vi "debug.vi"(9 "压力点个数":dbl, 10 "检定次数":dbl) -> (6 "I":dbl[](array[numeric]), 8 "A":dbl[](array[numeric]))   [LabVIEW 2017]
panel:
  in  "产品编号":string[](array[string])
  in  "参数计算":bool
  in  "加载参数":bool
  in  "保存参数":bool
  in  "偏置增益调试文件名":string="2022917_1556_70.0"
  in  "补偿电阻调试文件名":string="2022917_1556_70.0"
  in  "控制板调试":bool
  out "Rp":dbl[](array[numeric])
  out "Rs":dbl[](array[numeric])
  in  "退出":bool
  in  "行程测试":bool
  out "Rx":dbl[](array[numeric])
  out "Rf":dbl[](array[numeric])
  in  "偏置增益计算":bool
  in  "补偿电阻计算":bool
  out "理论曲线":string
  in  "理论偏置 b":dbl=200.0
  in  "理论放大 K":dbl=287.5
  out "Vx":dbl[](array[numeric])
  in  "Radj1":dbl[](array[numeric])
  in  "RG":dbl[](array[numeric])
  in  "R5-1":dbl[](array[numeric])
  in  "R4-6":dbl[](array[numeric])
  in  "R5-6":dbl[](array[numeric])
  in  "R5-5":dbl[](array[numeric])
  in  "R5-4":dbl[](array[numeric])
  in  "R4-4":dbl[](array[numeric])
  in  "R3-2":dbl[](array[numeric])
  in  "R3-1":dbl[](array[numeric])
  in  "数据":dbl[][](array[numeric])=[[199.921, 4.0, 7.8325, 4.0, -2.844e-06, -3.3e-06, -3.109e-06, -3.045e-06, -2.897e-06, 1.0, 0.0], [299.9351, 4.0, 7.8338, 1.0, -3.491e-06, -2.918e-06, -3.332e-06, -2.78e-06, -3.204e-06, 0.0, 0.0], [399.96, 4.0, 7.8346, -3.12e-06, -3.289e-06, -2.96e-06, -3.141e-06, -3.385e-06, -2.844e-06, 0.0, 0.0], [400.0285, -4.0, 7.8346, 0.0, -3.342e-06, -3.162e-06, -3.194e-06, -3.056e-06, -3.194e-06, 0.0, 0.0], [300.0653, -4.0, 7.8332, -3.342e-06, -3.321e-06, -3.013e-06, -3.311e-06, -3.3e-06, -3.162e-06, 0.0, 0.0], [200.0595, -4.0, 7.8346, -2.907e-06, -3.194e-06, -3.257e-06, -3.204e-06, -3.077e-06, -2.971e-06, 0.0, 0.0], [199.9466, 4.0, 8.8568, 5.0, -3.353e-06, -3.799e-06, -3.565e-06, -3.746e-06, -3.374e-06, 0.0, 0.0], [299.95, 4.0, 8.8574, -3.311e-06, -3.502e-06, -3.364e-06, -3.618e-06, -3.12e-06, -3.406e-06, 0.0, 0.0], [399.8962, 4.0, 8.8567, -3.756e-06, -3.83e-06, -3.427e-06, -3.597e-06, -3.777e-06, -3.576e-06, 0.0, 0.0], [399.9835, -4.0, 8.8567, 0.0, -3.289e-06, -3.12e-06, -3.502e-06, -3.427e-06, -3.353e-06, 0.0, 0.0], [299.9459, -4.0, 8.8552, -3.512e-06, -3.65e-06, -3.809e-06, -3.48e-06, -3.3e-06, -3.767e-06, 0.0, 0.0], [199.9841, -4.0, 8.8564, -3.629e-06, -3.608e-06, -3.767e-06, -3.639e-06, -3.417e-06, -3.406e-06, 0.0, 0.0], [200.0, 4.0, 0.0, 1.0, 0.0, 0.0, 0.0, 0.0, 0.0, 0.0, 0.0], [300.0, 4.0, 0.0, 2.0, 0.0, 0.0, 0.0, 0.0, 0.0, 0.0, 0.0], [400.0, 4.0, 0.0, 3.0, 0.0, 0.0, 0.0, 0.0, 0.0, 0.0, 0.0], [400.0, -4.0, 0.0, 20.0, 0.0, 0.0, 0.0, 0.0, 0.0, 0.0, 0.0], [300.0, -4.0, 0.0, 5.0, 0.0, 0.0, 0.0, 0.0, 0.0, 0.0, 0.0], [200.0, -4.0, 0.0, 6.0, 0.0, 0.0, 0.0, 0.0, 0.0, 0.0, 0.0], [200.0, 0.0, 0.0, 7.0, 0.0, 0.0, 0.0, 0.0, 0.0, 0.0, 0.0], [300.0, 0.0, 0.0, 8.0, 0.0, 0.0, 0.0, 0.0, 0.0, 0.0, 0.0], [400.0, 0.0, 0.0, 9.0, 0.0, 0.0, 0.0, 0.0, 0.0, 0.0, 0.0], [400.0, -7.0, 0.0, 10.0, 0.0, 0.0, 0.0, 0.0, 0.0, 0.0, 0.0], [300.0, -7.0, 0.0, 11.0, 0.0, 0.0, 0.0, 0.0, 0.0, 0.0, 0.0], [200.0, -7.0, 0.0, 12.0, 0.0, 0.0, 0.0, 0.0, 0.0, 0.0, 0.0], [0.0, 0.0, 0.0, 13.0, 0.0, 0.0, 0.0, 0.0, 0.0, 0.0, 0.0], [0.0, 0.0, 0.0, 14.0, 0.0, 0.0, 0.0, 0.0, 0.0, 0.0, 0.0], [0.0, 0.0, 0.0, 15.0, 0.0, 0.0, 0.0, 0.0, 0.0, 0.0, 0.0], [0.0, -7.0, 0.0, 16.0, 0.0, 0.0, 0.0, 0.0, 0.0, 0.0, 0.0], [0.0, -7.0, 0.0, 17.0, 0.0, 0.0, 0.0, 0.0, 0.0, 0.0, 0.0], [0.0, -7.0, 0.0, 18.0, 0.0, 0.0, 0.0, 0.0, 0.0, 0.0, 0.0], [0.0, 0.0, 0.0, 19.0, 0.0, 0.0, 0.0, 0.0, 0.0, 0.0, 0.0], [0.0, 0.0, 0.0, 20.0, 0.0, 0.0, 0.0, 0.0, 0.0, 0.0, 0.0], [0.0, 0.0, 0.0, 21.0, 0.0, 0.0, 0.0, 0.0, 0.0, 0.0, 0.0], [0.0, -7.0, 0.0, 22.0, 0.0, 0.0, 0.0, 0.0, 0.0, 0.0, 0.0], [0.0, -7.0, 0.0, 23.0, 0.0, 0.0, 0.0, 0.0, 0.0, 0.0, 0.0], [0.0, -7.0, 0.0, 24.0, 0.0, 0.0, 0.0, 0.0, 0.0, 0.0, 0.0], [0.0, 0.0, 0.0, 25.0, 0.0, 0.0, 0.0, 0.0, 0.0, 0.0, 0.0], [0.0, 0.0, 0.0, 26.0, 0.0, 0.0, 0.0, 0.0, 0.0, 0.0, 0.0], [0.0, 0.0, 0.0, 27.0, 0.0, 0.0, 0.0, 0.0, 0.0, 0.0, 0.0]]
  # "多通道 传感器调试系统"
  # "结果计算"
  # "参数设置  单位（Ω）"
  # "1"
  # "2"
  # "3"
  # "4"
  # "5"
  # "6"
  # "7"
  # "8"
  # "9"
  # "10"
  # "1"
  # "2"
  # "3"
  # "4"
  # "5"
  # "6"
  # "7"
  # "8"
  # "9"
  # "10"
  # "传感器编号"
  # "A"
  # "R3-1"
  # "I(mA)"
  # "R3-2"
  # "Vx(V)"
  # "R4-4"
  # "R4-6"
  # "Rs(kΩ)"
  # "R5-1"
  # "Rp(MΩ)"
  # "R5-4"
  # "R5-5"
  # "Rf(kΩ)"
  # "R5-6"
  # "Rx(Ω)"
  # "RG"
  # "Radj1"
  # "注意：\n调试系统，支持可变个传感器调试，不必连接10个。支持个数范围（1-无穷大）\n调试前，请参照调试规范，预先筛选安装并测量上述每个电阻的电阻值。\n在计算 补偿电阻 与 偏置增益 前 请按照说明规范设置参数，并进行相应的自动化测试。\n计算 补偿电阻 与 偏置增益 请输入正确的信息。如需 系统自动获取，请置空相应输入信息。\n补偿电阻调试时，请在低温（-40℃）与高温（70℃）两个温度点进行，压力点设置为常压、15MPa两个点。\n偏置增益调试时、请在常温下进行6个压力点(20KPa, 100KPa, 1000KPa, 5000KPa, 10000KPa, 15000KPa)的测量。"
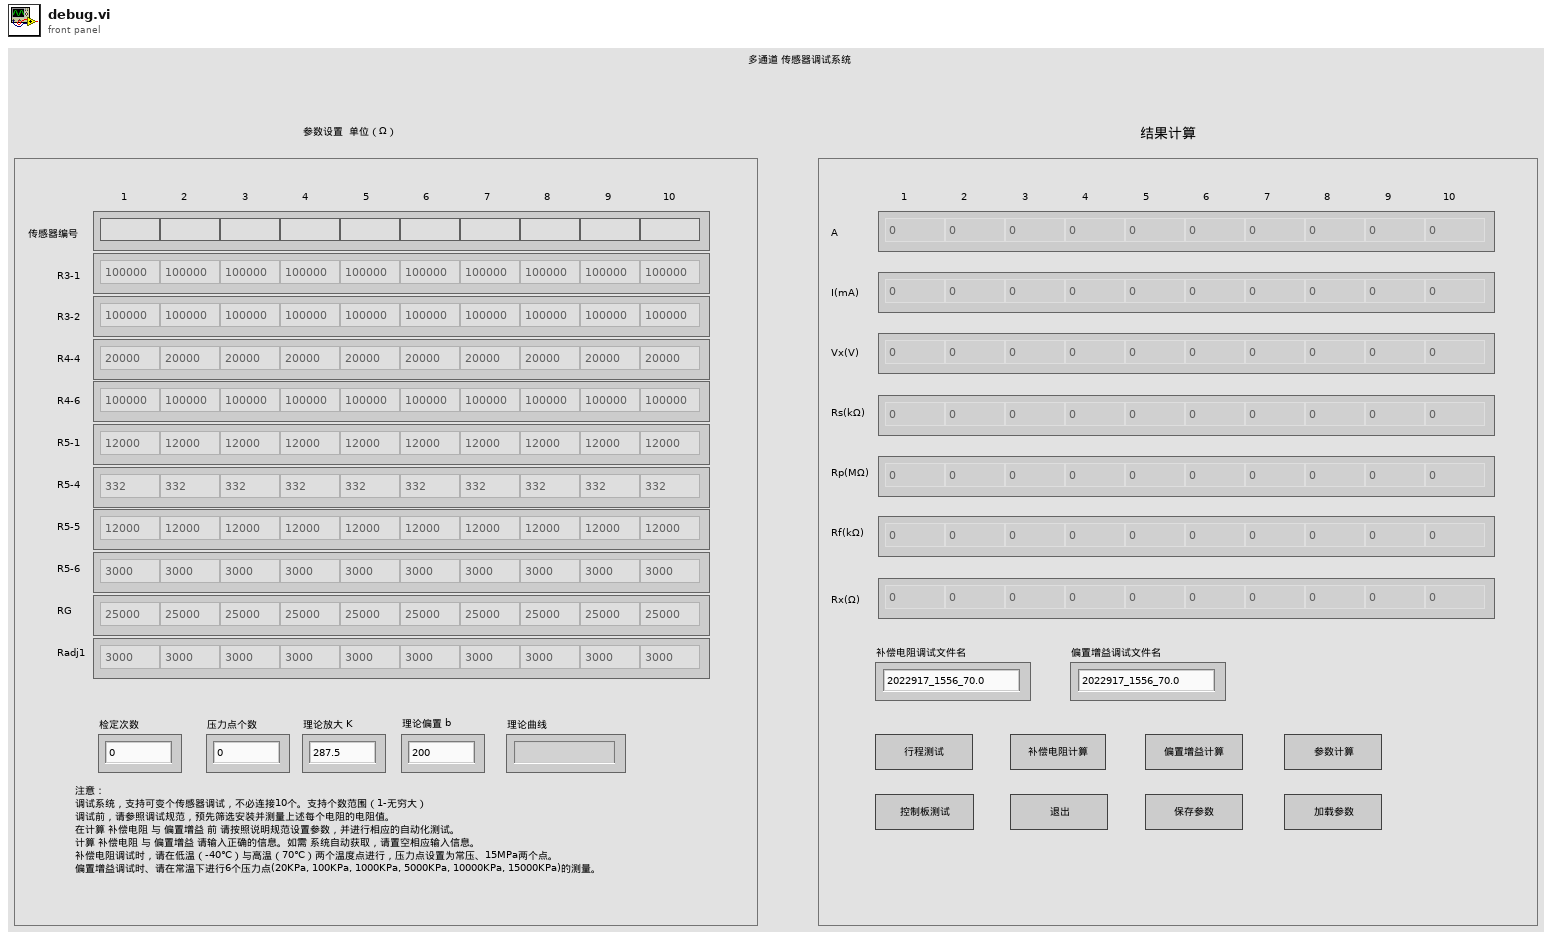
[diagram p1: front panel]
types:
  T1 = enum32{"Invalid", "Standard", "Closed", "Hidden", "Minimized", "Maximized"}
  T2 = enum16{"open", "replace", "create", "open or create", "replace or create", "replace or create with confirmation"}
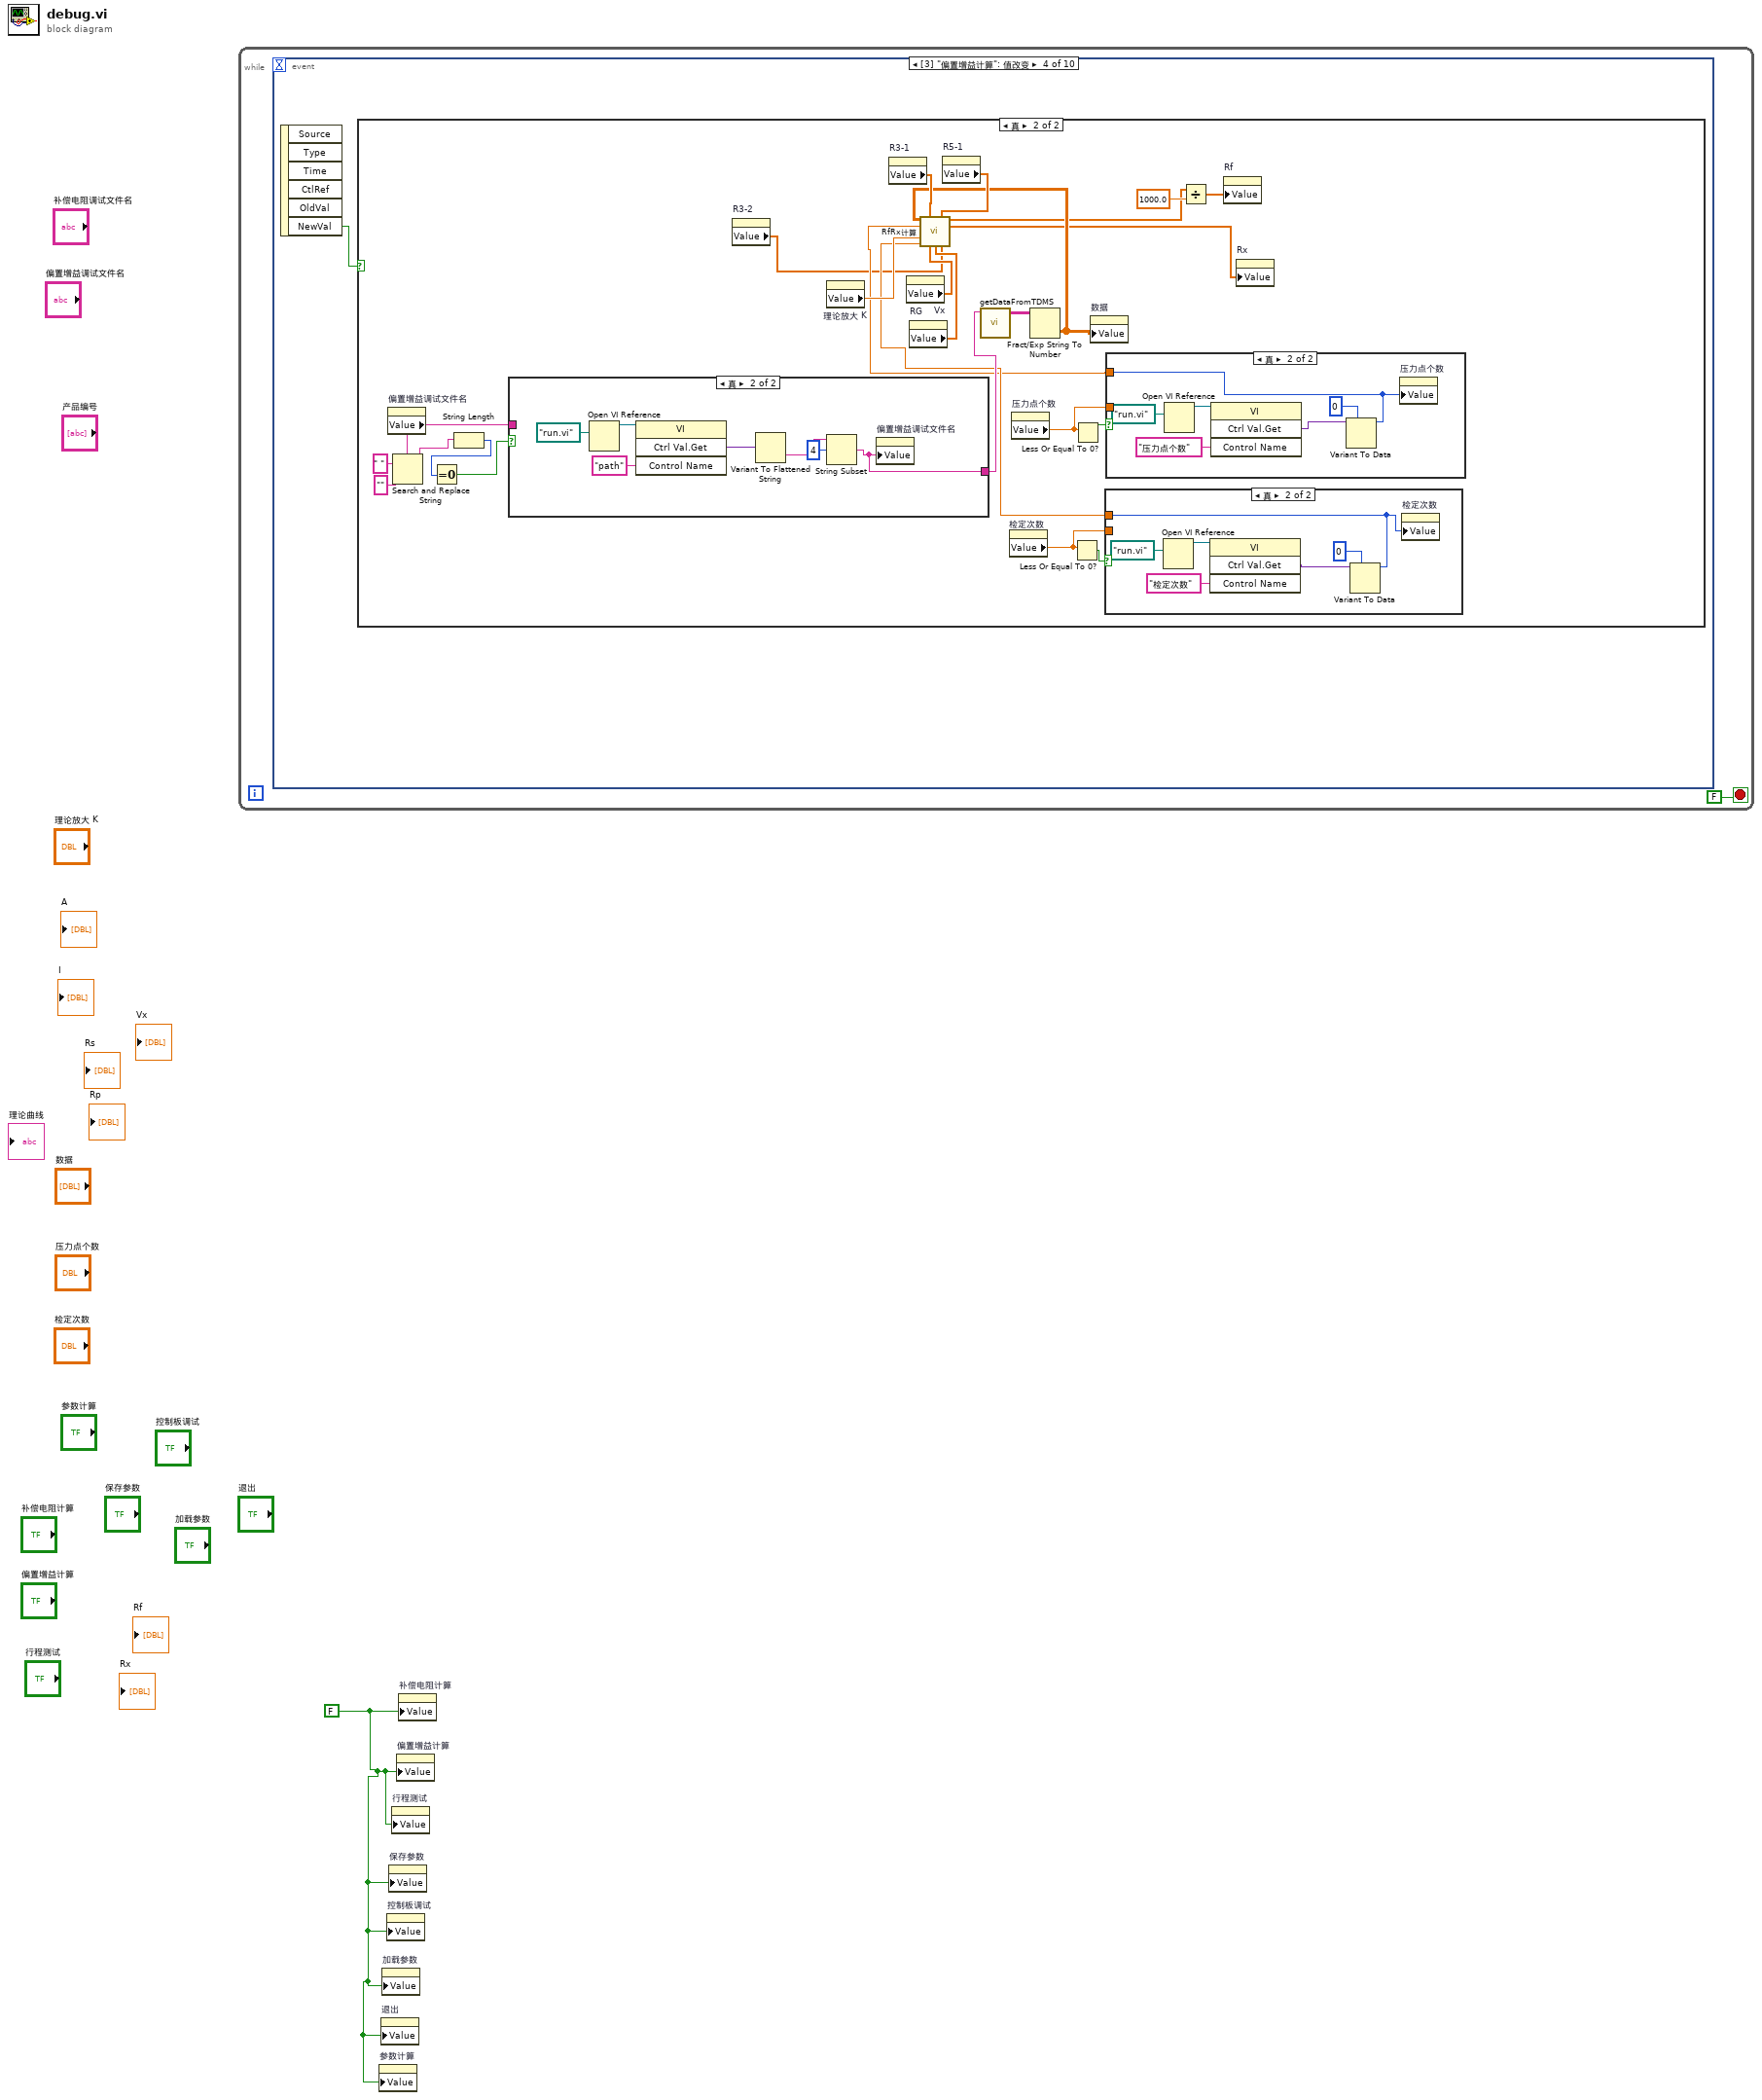
[diagram p0: block diagram]
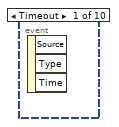
[diagram p2: hidden frame]
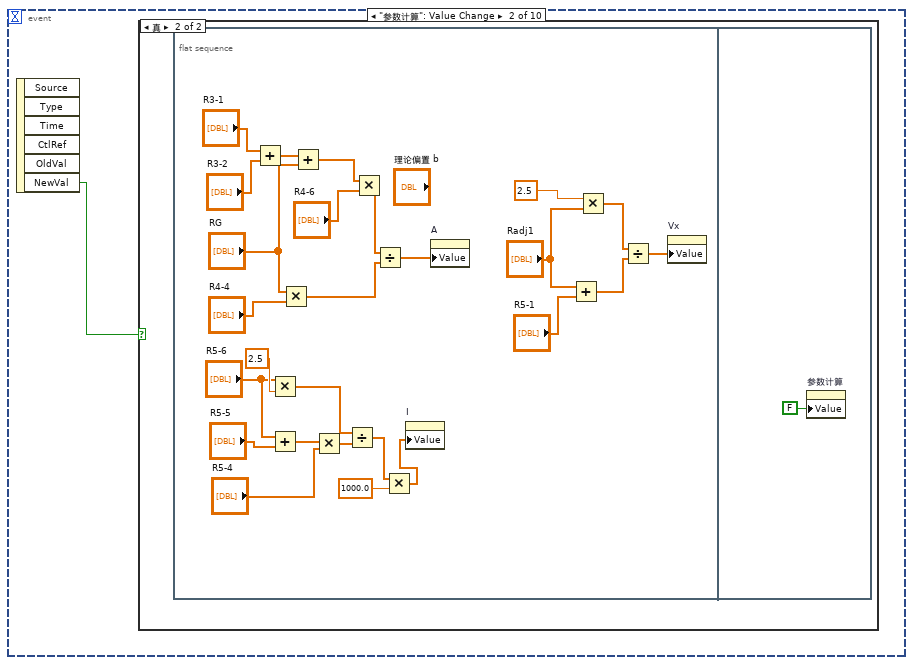
[diagram p3: hidden frame]
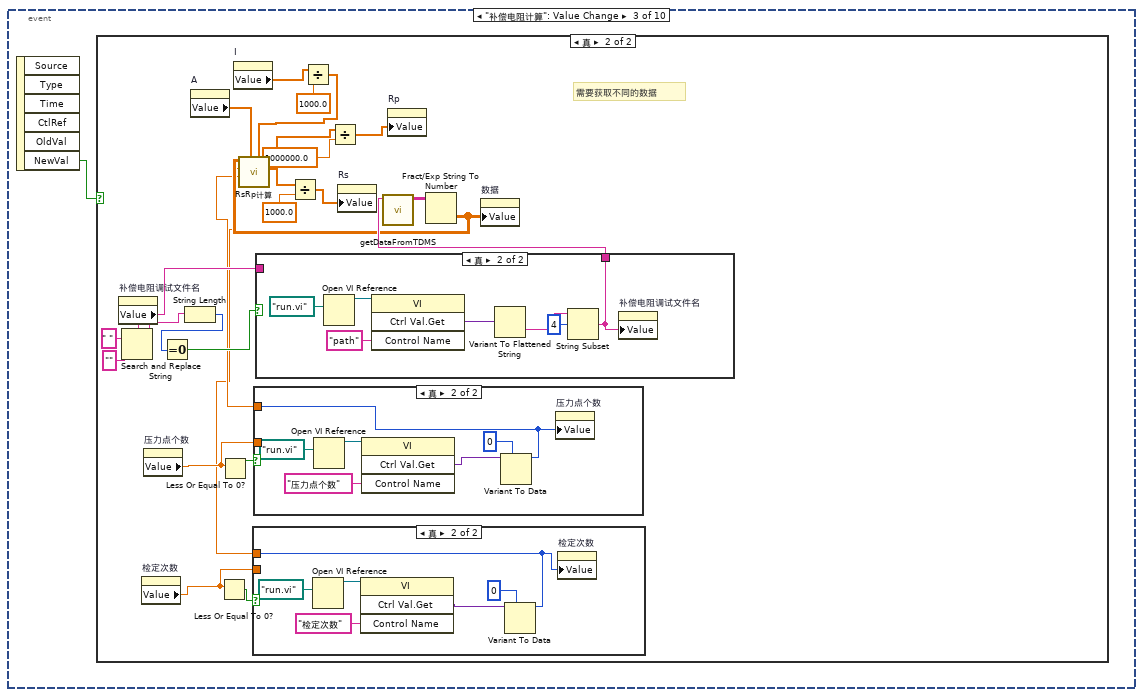
[diagram p5: hidden frame]
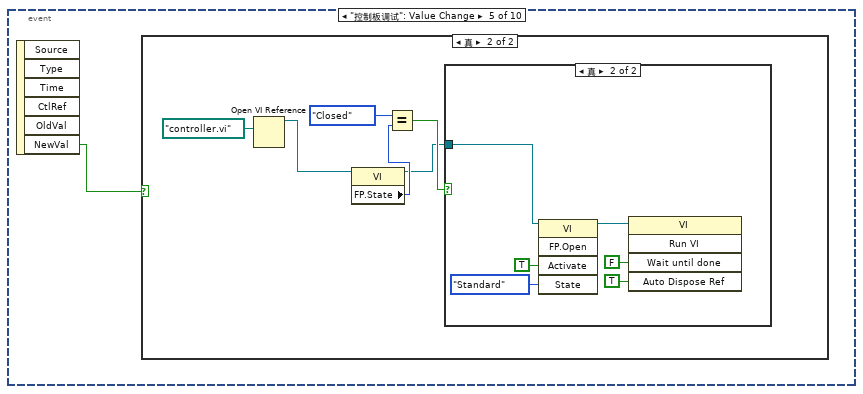
[diagram p14: hidden frame]
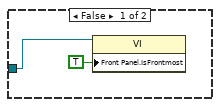
[diagram p16: hidden frame]
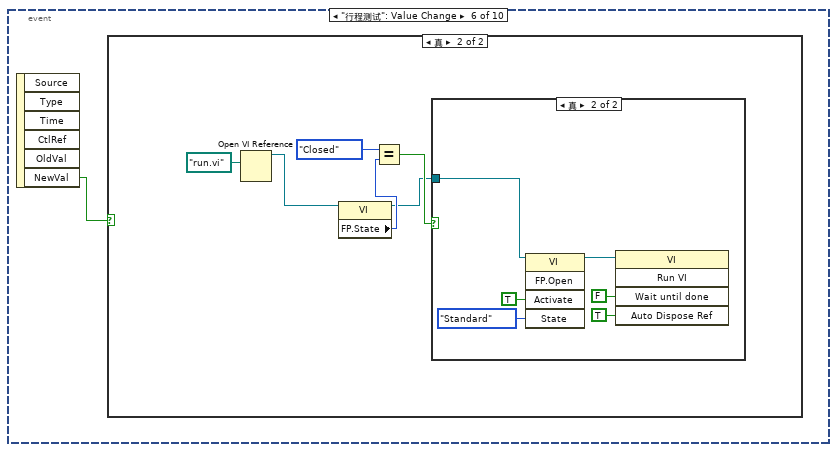
[diagram p17: hidden frame]
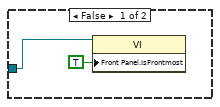
[diagram p19: hidden frame]
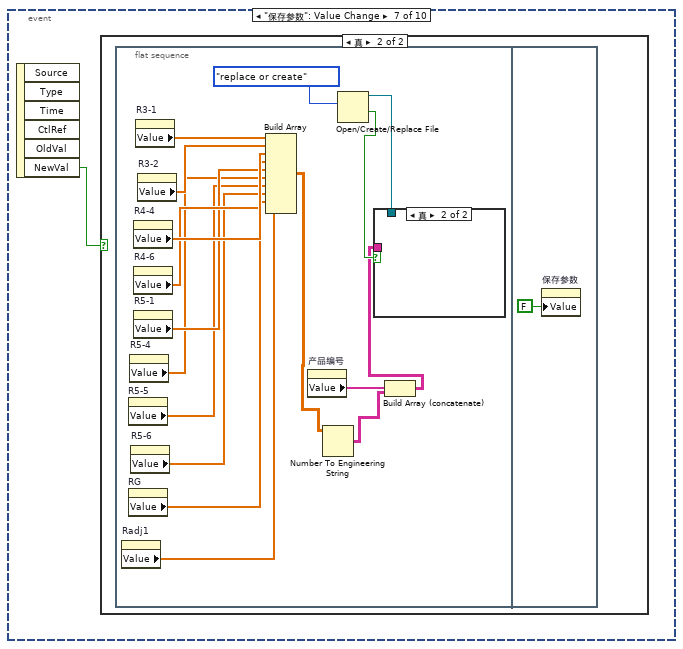
[diagram p20: hidden frame]
diagram:
  w1 = FALSE ("补偿电阻计算")
  n1 = while {
    stop <- FALSE stop-if-true
    n2 = event shown="[3] \"偏置增益计算\": 值改变" {
      selector: _ -> [_ _ _ _ _ _ _ _ _ _]
      dyn-events: _ -> [_ _ _ _ _ _ _ _ _ _]
      timeout: _ -> [_ _ _ _ _ _ _ _ _ _]
      event Timeout {
        n3 = event-data() -> ()  [unwired: 1 in, 3 out]
      }
      event "参数计算": Value Change {
        n4 = event-data() -> ("NewVal"=w3:bool)  [unwired: 1 in, 5 out]
        n5 = case shown="真" w3 {
          frame False {
          }
          frame True {
            n6 = flat-sequence {
              frame #0 {
                n7 = Add(x="R3-1", y="R3-2") -> (x+y=w27:dbl[])
                n8 = Multiply(x="R5-6", y=2.5) -> (x*y=w13:dbl[])
                n9 = Add(x="R5-6", y="R5-5") -> (x+y=w16:dbl[])
                n10 = Multiply(x="RG", y="R4-4") -> (x*y=w21:dbl[])
                n11 = Add(x=w27, y="RG") -> (x+y=w25:dbl[])
                n12 = Multiply(x=w16, y="R5-4") -> (x*y=w14:dbl[])
                n13 = Divide(x=w13, y=w14) -> (x/y=w4:dbl[])
                n14 = Multiply(x=w25, y="R4-6") -> (x*y=w22:dbl[])
                n15 = Divide(x=w22, y=w21) -> (x/y=w20:dbl[])
                n16 = Multiply(x=w4, y=1000.0) -> (x*y=w5:dbl[])
                n17 = property on="I" class="Arr (严格)"("Value"=w5) -> ()  [unwired: 2 in, 2 out]
                n18 = property on="A" class="Arr (严格)"("Value"=w20) -> ()  [unwired: 2 in, 2 out]
                n19 = Add(x="Radj1", y="R5-1") -> (x+y=w8:dbl[])
                n20 = Multiply(x=2.5, y="Radj1") -> (x*y=w9:dbl[])
                n21 = Divide(x=w9, y=w8) -> (x/y=w7:dbl[])
                n22 = property on="Vx" class="Arr (严格)"("Value"=w7) -> ()  [unwired: 2 in, 2 out]
              }
              frame #1 {
                n23 = property on="参数计算" class="Bool (严格)"("Value"=FALSE ("参数计算")) -> ()  [unwired: 2 in, 2 out]
              }
            }
          }
        }
      }
      event "补偿电阻计算": Value Change {
        n24 = event-data() -> ("NewVal"=w31:bool)  [unwired: 1 in, 5 out]
        n25 = case shown="真" w31 {
          frame False {
          }
          frame True {
            # "需要获取不同的数据"
            n26 = property on="补偿电阻调试文件名" class="Str"() -> ("Value"=w51:string)  [unwired: 2 in, 2 out]
            n27 = Search and Replace String(input string=w51, search string=" " ("搜索字符串"), replace string="" ("替换字符串(\"\")")) -> (result string=w52:string)  [unwired: 5 in, 3 out]
            n28 = property on="检定次数" class="DigNum (严格)"() -> ("Value"=w42:dbl)  [unwired: 2 in, 2 out]
            n29 = property on="压力点个数" class="DigNum (严格)"() -> ("Value"=w44:dbl)  [unwired: 2 in, 2 out]
            n30 = String Length(string=w52) -> (length=w56:i32)
            n31 = Equal To 0?(x=w56) -> (x = 0?=w55:bool)
            n32 = property on="A" class="Arr (严格)"() -> ("Value"=w47:dbl[])  [unwired: 2 in, 2 out]
            n33 = Less Or Equal To 0?(x=w42) -> (x <= 0?=w45:bool)
            n34 = Less Or Equal To 0?(x=w44) -> (x <= 0?=w46:bool)
            n35 = property on="I" class="Arr (严格)"() -> ("Value"=w34:dbl[])  [unwired: 2 in, 2 out]
            n36 = case shown="真" w45 {
              tunnel: [w57 w58] -> w41
              tunnel: w42 -> [w57 _]
              frame False {
              }
              frame True {
                n37 = Open VI Reference(vi path=path "run.vi" ("VI路径")) -> (vi reference=w62:refnum<vi>)  [unwired: 5 in, 1 out]
                n38 = invoke class="VI" method="Ctrl Val.Get"(reference=w62, "Control Name"="检定次数" ("控件名")) -> ("Get Control Value Variant"=w59:variant)  [unwired: 2 in, 3 out]
                n39 = Variant To Data(type=0, Variant=w59) -> (data=w58:i32)  [unwired: 1 in, 1 out]
                n40 = property on="检定次数" class="DigNum (严格)"("Value"=w58) -> ()  [unwired: 2 in, 2 out]
              }
            }
            n41 = case shown="真" w46 {
              tunnel: [w64 w65] -> w43
              tunnel: w44 -> [w64 _]
              frame False {
              }
              frame True {
                n42 = Open VI Reference(vi path=path "run.vi" ("VI路径")) -> (vi reference=w69:refnum<vi>)  [unwired: 5 in, 1 out]
                n43 = invoke class="VI" method="Ctrl Val.Get"(reference=w69, "Control Name"="压力点个数" ("控件名")) -> ("Get Control Value Variant"=w67:variant)  [unwired: 2 in, 3 out]
                n44 = Variant To Data(type=0, Variant=w67) -> (data=w65:i32)  [unwired: 1 in, 1 out]
                n45 = property on="压力点个数" class="DigNum (严格)"("Value"=w65) -> ()  [unwired: 2 in, 2 out]
              }
            }
            n46 = case shown="真" w55 {
              tunnel: [w71 w72] -> w50
              tunnel: w51 -> [w71 _]
              frame False {
              }
              frame True {
                n47 = Open VI Reference(vi path=path "run.vi" ("VI路径")) -> (vi reference=w77:refnum<vi>)  [unwired: 5 in, 1 out]
                n48 = invoke class="VI" method="Ctrl Val.Get"(reference=w77, "Control Name"="path" ("控件名")) -> ("Get Control Value Variant"=w75:variant)  [unwired: 2 in, 3 out]
                n49 = Variant To Flattened String(Variant=w75) -> (data string=w74:string)  [unwired: 1 out]
                n50 = String Subset(string=w74, offset (0)=4 ("偏移量(0)")) -> (substring=w72:string)  [unwired: 1 in]
                n51 = property on="补偿电阻调试文件名" class="Str"("Value"=w72) -> ()  [unwired: 2 in, 2 out]
              }
            }
            n52 = Divide(x=w34, y=1000.0) -> (x/y=w32:dbl[])
            n53 = call "getDataFromTDMS.vi"("文件名称"=w50) -> ("数据"=w49:string[][])  [unwired: 10 in]
            n54 = Fract/Exp String To Number(string=w49) -> (number=w48:dbl[][])  [unwired: 3 in, 1 out]
            n55 = call "RsRp计算.vi"("I"=w32, "A"=w47, "压力点个数"=w43, "检定次数"=w41, "数据"=w48) -> ("Rs"=w37:dbl[], "Rp"=w39:dbl[])  [unwired: 4 in, 1 out]
            n56 = Divide(x=w37, y=1000.0) -> (x/y=w36:dbl[])
            n57 = Divide(x=w39, y=1000000.0) -> (x/y=w40:dbl[])
            n58 = property on="Rs" class="Arr (严格)"("Value"=w36) -> ()  [unwired: 2 in, 2 out]
            n59 = property on="Rp" class="Arr (严格)"("Value"=w40) -> ()  [unwired: 2 in, 2 out]
            n60 = property on="数据" class="Arr (严格)"("Value"=w48) -> ()  [unwired: 2 in, 2 out]
          }
        }
      }
      event "偏置增益计算": Value Change {
        n61 = event-data() -> ("NewVal"=w79:bool)  [unwired: 1 in, 5 out]
        n62 = case shown="真" w79 {
          frame False {
          }
          frame True {
            n63 = property on="偏置增益调试文件名" class="Str"() -> ("Value"=w94:string)  [unwired: 2 in, 2 out]
            n64 = Search and Replace String(input string=w94, search string=" " ("搜索字符串"), replace string="" ("替换字符串(\"\")")) -> (result string=w96:string)  [unwired: 5 in, 3 out]
            n65 = String Length(string=w96) -> (length=w99:i32)
            n66 = Equal To 0?(x=w99) -> (x = 0?=w95:bool)
            n67 = case shown="真" w95 {
              tunnel: [w119 w120] -> w93
              tunnel: w94 -> [w119 _]
              frame False {
              }
              frame True {
                n68 = Open VI Reference(vi path=path "run.vi" ("VI路径")) -> (vi reference=w125:refnum<vi>)  [unwired: 5 in, 1 out]
                n69 = invoke class="VI" method="Ctrl Val.Get"(reference=w125, "Control Name"="path" ("控件名")) -> ("Get Control Value Variant"=w123:variant)  [unwired: 2 in, 3 out]
                n70 = Variant To Flattened String(Variant=w123) -> (data string=w122:string)  [unwired: 1 out]
                n71 = String Subset(string=w122, offset (0)=4 ("偏移量(0)")) -> (substring=w120:string)  [unwired: 1 in]
                n72 = property on="偏置增益调试文件名" class="Str"("Value"=w120) -> ()  [unwired: 2 in, 2 out]
              }
            }
            n73 = property on="R3-2" class="Arr (严格)"() -> ("Value"=w84:dbl[])  [unwired: 2 in, 2 out]
            n74 = property on="理论放大 K" class="DigNum (严格)"() -> ("Value"=w104:dbl)  [unwired: 2 in, 2 out]
            n75 = property on="R3-1" class="Arr (严格)"() -> ("Value"=w103:dbl[])  [unwired: 2 in, 2 out]
            n76 = property on="Vx" class="Arr (严格)"() -> ("Value"=w101:dbl[])  [unwired: 2 in, 2 out]
            n77 = property on="RG" class="Arr (严格)"() -> ("Value"=w100:dbl[])  [unwired: 2 in, 2 out]
            n78 = property on="R5-1" class="Arr (严格)"() -> ("Value"=w102:dbl[])  [unwired: 2 in, 2 out]
            n79 = call "getDataFromTDMS.vi"("文件名称"=w93) -> ("数据"=w92:string[][])  [unwired: 10 in]
            n80 = property on="检定次数" class="DigNum (严格)"() -> ("Value"=w86:dbl)  [unwired: 2 in, 2 out]
            n81 = property on="压力点个数" class="DigNum (严格)"() -> ("Value"=w85:dbl)  [unwired: 2 in, 2 out]
            n82 = Fract/Exp String To Number(string=w92) -> (number=w91:dbl[][])  [unwired: 3 in, 1 out]
            n83 = Less Or Equal To 0?(x=w86) -> (x <= 0?=w89:bool)
            n84 = Less Or Equal To 0?(x=w85) -> (x <= 0?=w90:bool)
            n85 = property on="数据" class="Arr (严格)"("Value"=w91) -> ()  [unwired: 2 in, 2 out]
            n86 = case shown="真" w89 {
              tunnel: [w105 w106] -> w88
              tunnel: w86 -> [w105 _]
              frame False {
              }
              frame True {
                n87 = Open VI Reference(vi path=path "run.vi" ("VI路径")) -> (vi reference=w110:refnum<vi>)  [unwired: 5 in, 1 out]
                n88 = invoke class="VI" method="Ctrl Val.Get"(reference=w110, "Control Name"="检定次数" ("控件名")) -> ("Get Control Value Variant"=w107:variant)  [unwired: 2 in, 3 out]
                n89 = Variant To Data(type=0, Variant=w107) -> (data=w106:i32)  [unwired: 1 in, 1 out]
                n90 = property on="检定次数" class="DigNum (严格)"("Value"=w106) -> ()  [unwired: 2 in, 2 out]
              }
            }
            n91 = case shown="真" w90 {
              tunnel: [w112 w113] -> w87
              tunnel: w85 -> [w112 _]
              frame False {
              }
              frame True {
                n92 = Open VI Reference(vi path=path "run.vi" ("VI路径")) -> (vi reference=w117:refnum<vi>)  [unwired: 5 in, 1 out]
                n93 = invoke class="VI" method="Ctrl Val.Get"(reference=w117, "Control Name"="压力点个数" ("控件名")) -> ("Get Control Value Variant"=w115:variant)  [unwired: 2 in, 3 out]
                n94 = Variant To Data(type=0, Variant=w115) -> (data=w113:i32)  [unwired: 1 in, 1 out]
                n95 = property on="压力点个数" class="DigNum (严格)"("Value"=w113) -> ()  [unwired: 2 in, 2 out]
              }
            }
            n96 = call "RfRx计算.vi"("输入数据"=w91, "R3-1"=w103, "R5-1"=w102, "压力点个数"=w87, "理论K"=w104, "检定次数"=w88, "Vx"=w101, "RG"=w100, "R3-2"=w84) -> ("Rf"=w81:dbl[], "Rx"=w80:dbl[])  [unwired: 5 in]
            n97 = Divide(x=w81, y=1000.0) -> (x/y=w82:dbl[])
            n98 = property on="Rf" class="Arr (严格)"("Value"=w82) -> ()  [unwired: 2 in, 2 out]
            n99 = property on="Rx" class="Arr (严格)"("Value"=w80) -> ()  [unwired: 2 in, 2 out]
          }
        }
      }
      event "控制板调试": Value Change {
        n100 = event-data() -> ("NewVal"=w127:bool)  [unwired: 1 in, 5 out]
        n101 = case shown="真" w127 {
          frame False {
          }
          frame True {
            n102 = Open VI Reference(vi path=path "controller.vi" ("VI路径")) -> (vi reference=w128:refnum<vi>)  [unwired: 5 in, 1 out]
            n103 = property class="VI"(reference=w128) -> (reference out=w129:refnum<vi>, "FP.State"=w132:T1)  [unwired: 1 in, 1 out]
            n104 = Equal?(x=T1."Closed", y=w132) -> (x = y?=w130:bool)
            n105 = case shown="真" w130 {
              tunnel: w129 -> [w134 w136]
              frame False {
                n106 = property class="VI"(reference=w134, "Front Panel.IsFrontmost"=TRUE ("前面板窗口:在最前")) -> ()  [unwired: 1 in, 2 out]
              }
              frame True {
                n107 = invoke class="VI" method="FP.Open"(reference=w136, "Activate"=TRUE ("激活？"), "State"=T1."Standard" ("状态")) -> (reference out=w139:refnum<vi>)  [unwired: 2 in, 4 out]
                n108 = invoke class="VI" method="Run VI"(reference=w139, "Wait until done"=FALSE ("结束前等待"), "Auto Dispose Ref"=TRUE ("自动销毁引用")) -> ()  [unwired: 2 in, 5 out]
              }
            }
          }
        }
      }
      event "行程测试": Value Change {
        n109 = event-data() -> ("NewVal"=w142:bool)  [unwired: 1 in, 5 out]
        n110 = case shown="真" w142 {
          frame False {
          }
          frame True {
            n111 = Open VI Reference(vi path=path "run.vi" ("VI路径")) -> (vi reference=w143:refnum<vi>)  [unwired: 5 in, 1 out]
            n112 = property class="VI"(reference=w143) -> (reference out=w144:refnum<vi>, "FP.State"=w147:T1)  [unwired: 1 in, 1 out]
            n113 = Equal?(x=T1."Closed", y=w147) -> (x = y?=w145:bool)
            n114 = case shown="真" w145 {
              tunnel: w144 -> [w149 w151]
              frame False {
                n115 = property class="VI"(reference=w149, "Front Panel.IsFrontmost"=TRUE ("前面板窗口:在最前")) -> ()  [unwired: 1 in, 2 out]
              }
              frame True {
                n116 = invoke class="VI" method="FP.Open"(reference=w151, "Activate"=TRUE ("激活？"), "State"=T1."Standard" ("状态")) -> (reference out=w154:refnum<vi>)  [unwired: 2 in, 4 out]
                n117 = invoke class="VI" method="Run VI"(reference=w154, "Wait until done"=FALSE ("结束前等待"), "Auto Dispose Ref"=TRUE ("自动销毁引用")) -> ()  [unwired: 2 in, 5 out]
              }
            }
          }
        }
      }
      event "保存参数": Value Change {
        n118 = event-data() -> ("NewVal"=w157:bool)  [unwired: 1 in, 5 out]
        n119 = case shown="真" w157 {
          frame False {
          }
          frame True {
            n120 = flat-sequence {
              frame #0 {
                n121 = property on="Radj1" class="Arr (严格)"() -> ("Value"=w160:dbl[])  [unwired: 2 in, 2 out]
                n122 = property on="R5-5" class="Arr (严格)"() -> ("Value"=w168:dbl[])  [unwired: 2 in, 2 out]
                n123 = property on="RG" class="Arr (严格)"() -> ("Value"=w166:dbl[])  [unwired: 2 in, 2 out]
                n124 = property on="R5-4" class="Arr (严格)"() -> ("Value"=w169:dbl[])  [unwired: 2 in, 2 out]
                n125 = property on="R5-6" class="Arr (严格)"() -> ("Value"=w167:dbl[])  [unwired: 2 in, 2 out]
                n126 = property on="R4-4" class="Arr (严格)"() -> ("Value"=w172:dbl[])  [unwired: 2 in, 2 out]
                n127 = property on="R4-6" class="Arr (严格)"() -> ("Value"=w171:dbl[])  [unwired: 2 in, 2 out]
                n128 = property on="R5-1" class="Arr (严格)"() -> ("Value"=w170:dbl[])  [unwired: 2 in, 2 out]
                n129 = property on="R3-1" class="Arr (严格)"() -> ("Value"=w174:dbl[])  [unwired: 2 in, 2 out]
                n130 = property on="R3-2" class="Arr (严格)"() -> ("Value"=w173:dbl[])  [unwired: 2 in, 2 out]
                n131 = Build Array(w174, w173, w172, w171, w170, w169, w168, w167, w166, w160) -> (w158:dbl[][])
                n132 = property on="产品编号" class="Arr (严格)"() -> ("Value"=w162:string[])  [unwired: 2 in, 2 out]
                n133 = Number To Engineering String(4:w158) -> (0:w159:string[][])  [unwired: 3 in]
                n134 = Open/Create/Replace File(operation (0:open)=T2."replace or create" ("操作(0:open)")) -> (refnum out=w163:refnum<file>, cancelled=w164:bool)  [unwired: 5 in, 1 out]
                n135 = Build Array (concatenate)(w162, w159) -> (w161:string[][])
                n136 = case shown="真" w164 {
                  tunnel: w161 -> [w176 _]
                  tunnel: w163 -> [w175 _]
                  frame False {
                    n137 = Write to Binary File(file (use dialog)=w175, data=w176) -> (refnum out=w177:refnum<file>)  [unwired: 4 in, 2 out]
                    n138 = Close File(refnum=w177) -> ()  [unwired: 1 in, 2 out]
                  }
                  frame True {
                  }
                }
              }
              frame #1 {
                n139 = property on="保存参数" class="Bool (严格)"("Value"=FALSE ("保存参数")) -> ()  [unwired: 2 in, 2 out]
              }
            }
          }
        }
      }
      event "加载参数": Value Change {
        n140 = event-data() -> ("NewVal"=w179:bool)  [unwired: 1 in, 5 out]
        n141 = case shown="真" w179 {
          frame False {
          }
          frame True {
            n142 = flat-sequence {
              frame #0 {
                n143 = Open/Create/Replace File() -> (refnum out=w209:refnum<file>, error out=w210:errorcluster)  [unwired: 6 in, 1 out]
                n144 = Read from Binary File(5:string[][] [], 8:w210, 11:w209) -> (0:w207:errorcluster, 2:w184:string[][], 3:w208:refnum<file>)  [unwired: 3 in, 1 out]
                n145 = Index Array(array=w184, index (row)=0 ("索引 (行)")) -> (element=w185:string[])  [unwired: 1 in]
                n146 = Array Subset(array=w184, index (row)=1 ("索引")) -> (w180:string[][])  [unwired: 3 in]
                n147 = Fract/Exp String To Number(string=w180) -> (number=w181:dbl[][])  [unwired: 3 in, 1 out]
                n148 = property on="产品编号" class="Arr (严格)"("Value"=w185) -> ()  [unwired: 2 in, 2 out]
                n149 = Index Array(array=w181, index (row)=0 ("索引")) -> (element=w196:dbl[])  [unwired: 1 in]
                n150 = Index Array(array=w181, index (row)=6 ("索引")) -> (element=w190:dbl[])  [unwired: 1 in]
                n151 = Index Array(array=w181, index (row)=7 ("索引")) -> (element=w189:dbl[])  [unwired: 1 in]
                n152 = Index Array(array=w181, index (row)=8 ("索引")) -> (element=w188:dbl[])  [unwired: 1 in]
                n153 = Index Array(array=w181, index (row)=1 ("索引")) -> (element=w195:dbl[])  [unwired: 1 in]
                n154 = Index Array(array=w181, index (row)=3 ("索引")) -> (element=w193:dbl[])  [unwired: 1 in]
                n155 = Index Array(array=w181, index (row)=4 ("索引")) -> (element=w192:dbl[])  [unwired: 1 in]
                n156 = Index Array(array=w181, index (row)=5 ("索引")) -> (element=w191:dbl[])  [unwired: 1 in]
                n157 = Index Array(array=w181, index (row)=9 ("索引")) -> (element=w187:dbl[])  [unwired: 1 in]
                n158 = Index Array(array=w181, index (row)=2 ("索引")) -> (element=w194:dbl[])  [unwired: 1 in]
                n159 = Close File(refnum=w208, error in=w207) -> ()  [unwired: 2 out]
                n160 = property on="Radj1" class="Arr (严格)"("Value"=w187) -> ()  [unwired: 2 in, 2 out]
                n161 = property on="R5-5" class="Arr (严格)"("Value"=w190) -> ()  [unwired: 2 in, 2 out]
                n162 = property on="RG" class="Arr (严格)"("Value"=w188) -> ()  [unwired: 2 in, 2 out]
                n163 = property on="R5-4" class="Arr (严格)"("Value"=w191) -> ()  [unwired: 2 in, 2 out]
                n164 = property on="R5-6" class="Arr (严格)"("Value"=w189) -> ()  [unwired: 2 in, 2 out]
                n165 = property on="R4-4" class="Arr (严格)"("Value"=w194) -> ()  [unwired: 2 in, 2 out]
                n166 = property on="R4-6" class="Arr (严格)"("Value"=w193) -> ()  [unwired: 2 in, 2 out]
                n167 = property on="R5-1" class="Arr (严格)"("Value"=w192) -> ()  [unwired: 2 in, 2 out]
                n168 = property on="R3-1" class="Arr (严格)"("Value"=w196) -> ()  [unwired: 2 in, 2 out]
                n169 = property on="R3-2" class="Arr (严格)"("Value"=w195) -> ()  [unwired: 2 in, 2 out]
              }
              frame #1 {
                n170 = property on="加载参数" class="Bool (严格)"("Value"=FALSE ("加载参数")) -> ()  [unwired: 2 in, 2 out]
              }
            }
          }
        }
      }
      event "退出": Value Change {
        n171 = event-data() -> ("NewVal"=w212:bool)  [unwired: 1 in, 5 out]
        n172 = case shown="真" w212 {
          frame False {
          }
          frame True {
            n173 = flat-sequence {
              tunnel: [w216] -> w214
              frame #0 {
                n174 = property on="退出" class="Bool (严格)"("Value"=FALSE ("退出")) -> ()  [unwired: 2 in, 2 out]
              }
              frame #1 {
                n175 = control-ref of="本VI"() -> (w216:refnum<vi>)
              }
            }
            n176 = invoke class="VI" method="FP.Close"(reference=w214) -> (reference out=w213:refnum<vi>)  [unwired: 2 in, 2 out]
            n177 = invoke class="VI" method="Abort VI"(reference=w213) -> ()  [unwired: 2 in, 3 out]
          }
        }
      }
      event Panel Close {
        n178 = event-data() -> ()  [unwired: 1 in, 4 out]
        n179 = flat-sequence {
          tunnel: [w219] -> w217
          frame #0 {
            n180 = property on="退出" class="Bool (严格)"("Value"=FALSE ("退出")) -> ()  [unwired: 2 in, 2 out]
          }
          frame #1 {
            n181 = control-ref of="本VI"() -> (w219:refnum<vi>)
          }
        }
        n182 = invoke class="VI" method="Abort VI"(reference=w217) -> ()  [unwired: 2 in, 3 out]
      }
    }
  }
  n183 = property on="参数计算" class="Bool (严格)"("Value"=w1) -> ()  [unwired: 2 in, 2 out]
  n184 = property on="退出" class="Bool (严格)"("Value"=w1) -> ()  [unwired: 2 in, 2 out]
  n185 = property on="加载参数" class="Bool (严格)"("Value"=w1) -> ()  [unwired: 2 in, 2 out]
  n186 = property on="控制板调试" class="Bool (严格)"("Value"=w1) -> ()  [unwired: 2 in, 2 out]
  n187 = property on="保存参数" class="Bool (严格)"("Value"=w1) -> ()  [unwired: 2 in, 2 out]
  n188 = property on="行程测试" class="Bool (严格)"("Value"=w1) -> ()  [unwired: 2 in, 2 out]
  n189 = property on="偏置增益计算" class="Bool (严格)"("Value"=w1) -> ()  [unwired: 2 in, 2 out]
  n190 = property on="补偿电阻计算" class="Bool (严格)"("Value"=w1) -> ()  [unwired: 2 in, 2 out]
